vi "TSM SSC Digital Write Source Waveform [Site Unique].vi"(0 "Digital - Sessions in":T1, 1 "Waveform Name":string, 5 "Per-Site Waveforms":u32[][](array[numeric]) format="%.0x", 7 "Expand to Minimum Size?":bool caption="Expand to Minimum Size? (F)", 9 "Minimum Size":i32=128 caption="Minimum Size (128)", 11 "error in":errorcluster) -> (4 "Digital - Sessions out":T1, 15 "error out":errorcluster)   [LabVIEW 2019]
doc: "Writes one waveform per site after a waveform is created. Use this VI if you set the data mapping parameter of your source waveform to Site Unique. This VI accepts an array of per-site waveforms, where rows correspond to sites and columns correspond to samples."
uses:
  TSM/TSM SSC Digital.ctl
  <vilib>/NI_TestStand_SemiconductorModule/NI_TestStand_Semiconductor_Module.lvlibp/PinMap/Digital Pattern/PinQueryContext/DigitalPatternPinQueryContext.lvclass
  SSC Digital/SSC Digital.ctl
  bef7b3b5-9f14-4908-89fb-aa42e7d738f0.vi
  Shared SubVIs/Site List to Site Numbers.vi
  Shared SubVIs/Trim Whitespace [Inlined].vi
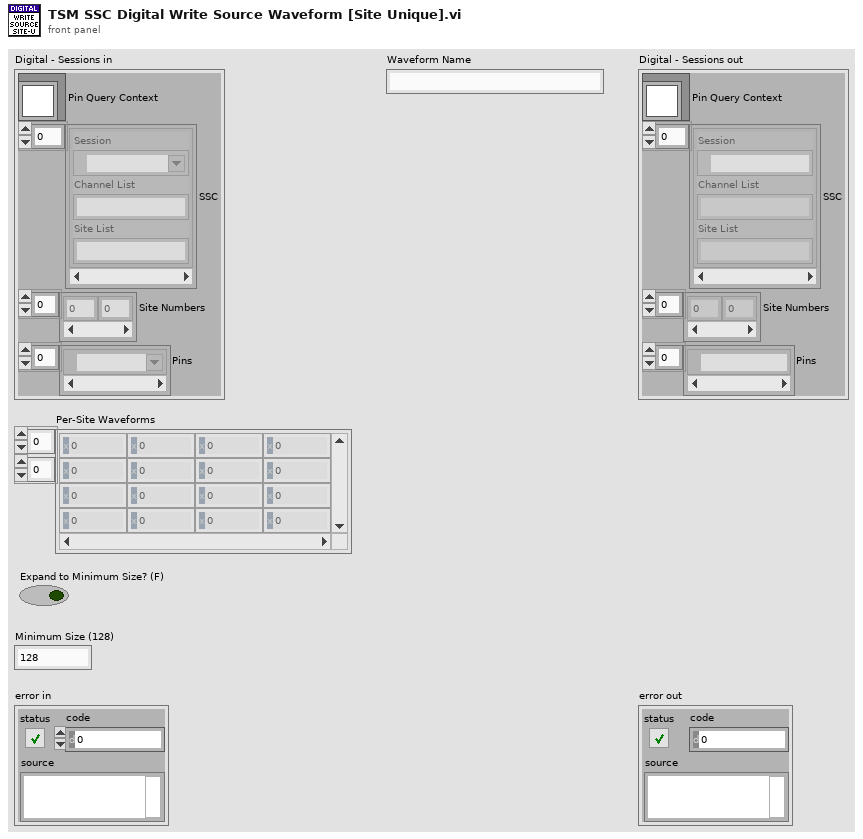
[diagram p1: front panel]
types:
  T1 = typedef "TSM SSC Digital.ctl" = cluster{"Pin Query Context":refnum<class "DigitalPatternPinQueryContext.lvclass">, "SSC":T2[], "Site Numbers":i32[], "Pins":tag[]}
  T2 = typedef "SSC Digital.ctl" = cluster{"Session":refnum<k15>, "Channel List":string, "Site List":string}
  T3 = typedef "Digital 2D Location.ctl" = cluster{"Row":i32, "Col":i32}
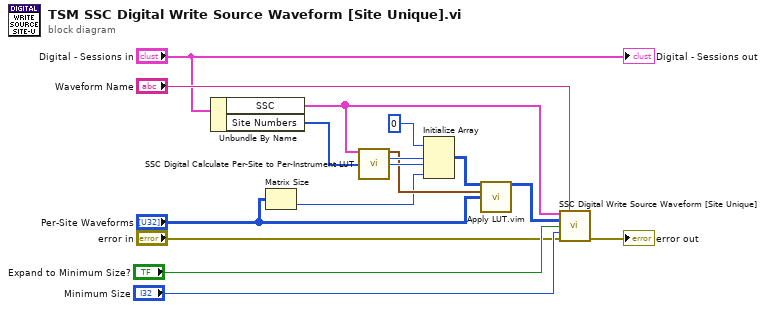
[diagram p0: block diagram]
diagram:
  n1 = Unbundle By Name("Digital - Sessions in") -> ("SSC"=w11:T2[], "Site Numbers"=w10:i32[])
  n2 = Matrix Size(0:"Per-Site Waveforms") -> (2:w1:i32)  [unwired: 1 out]
  n3 = call "SSC Digital Calculate Per-Site to Per-Instrument LUT.vi"("Digital SSC In"=w11, "Sites"=w10) -> ("Per-Site to Per-Instrument LUT"=w3:T3[], "Instrument Count"=w8:i32, "Max Sites on Instrument"=w9:i32)  [unwired: 11 in]
  n4 = Initialize Array(u32 0 ("element"), w8, w9, w1) -> (w4:u32[][][])
  n5 = call "Apply LUT.vim"("Initialized Array"=w4, "LUT"=w3, "Results to Apply LUT to"="Per-Site Waveforms") -> ("Array Out"=w5:u32[][][])  [unwired: 12 in]
  n6 = call "SSC Digital Write Source Waveform [Site Unique].vi"("Digital SSC in"=w11, "Waveform Name"="Waveform Name", "Per-Instrument Waveforms"=w5, "Expand to Minimum Size?"="Expand to Minimum Size?", "Minimum Size"="Minimum Size", "error in"="error in") -> ("error out"=→"error out":errorcluster)  [unwired: 8 in, 1 out]
  "Digital - Sessions out" <- "Digital - Sessions in"
